vi "IMAQ FPGA Camera Link Data to Pixels 8 Tap 10-Bit.vi"(1 "Camera Link Data":T1) -> (0 "Pixels":u16[](array[numeric]))   [LabVIEW 2020]
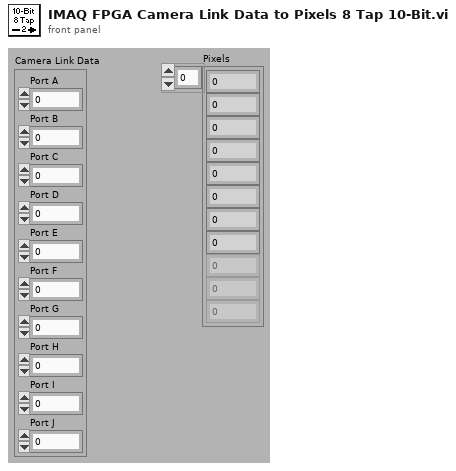
[diagram p1: front panel]
types:
  T1 = cluster{"Port A":u8, "Port B":u8, "Port C":u8, "Port D":u8, "Port E":u8, "Port F":u8, "Port G":u8, "Port H":u8, "Port I":u8, "Port J":u8}
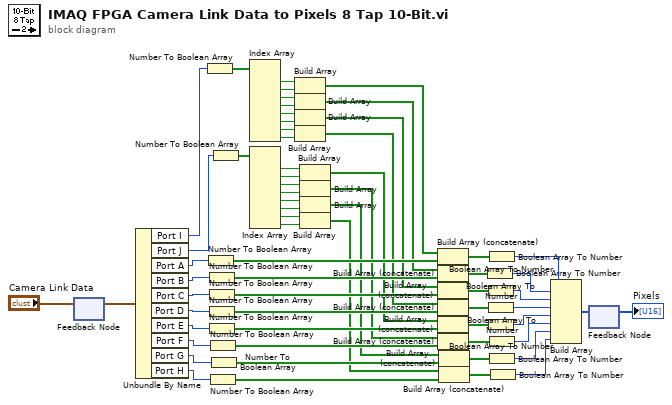
[diagram p0: block diagram]
diagram:
  n1 = feedback #1() -> (w1:T1)  [unwired: 1 in]
  n2 = feedback-in #1("Camera Link Data") -> ()
  n3 = Unbundle By Name(w1) -> ("Port I"=w52:u8, "Port J"=w51:u8, "Port A"=w64:u8, "Port B"=w61:u8, "Port C"=w58:u8, "Port D"=w56:u8, "Port E"=w49:u8, "Port F"=w47:u8, "Port G"=w18:u8, "Port H"=w7:u8)
  n4 = Number To Boolean Array(number=w52) -> (Boolean array=w40:bool[])
  n5 = Number To Boolean Array(number=w64) -> (Boolean array=w63:bool[])
  n6 = Number To Boolean Array(number=w61) -> (Boolean array=w60:bool[])
  n7 = Number To Boolean Array(number=w58) -> (Boolean array=w57:bool[])
  n8 = Number To Boolean Array(number=w56) -> (Boolean array=w55:bool[])
  n9 = Number To Boolean Array(number=w49) -> (Boolean array=w48:bool[])
  n10 = Number To Boolean Array(number=w47) -> (Boolean array=w26:bool[])
  n11 = Number To Boolean Array(number=w7) -> (Boolean array=w6:bool[])
  n12 = Number To Boolean Array(number=w18) -> (Boolean array=w14:bool[])
  n13 = Number To Boolean Array(number=w51) -> (Boolean array=w50:bool[])
  n14 = Index Array(array=w40) -> (element #1=w46:bool, element #2=w45:bool, element #3=w43:bool, element #4=w42:bool, element #5=w39:bool, element #6=w38:bool, element #7=w36:bool, element #8=w35:bool)  [unwired: 8 in]
  n15 = Index Array(array=w50) -> (element #1=w33:bool, element #2=w32:bool, element #3=w29:bool, element #4=w28:bool, element #5=w17:bool, element #6=w16:bool, element #7=w10:bool, element #8=w9:bool)  [unwired: 8 in]
  n16 = Build Array(w46, w45) -> (w44:bool[])
  n17 = Build Array(w43, w42) -> (w41:bool[])
  n18 = Build Array(w39, w38) -> (w37:bool[])
  n19 = Build Array(w36, w35) -> (w34:bool[])
  n20 = Build Array(w33, w32) -> (w31:bool[])
  n21 = Build Array(w29, w28) -> (w27:bool[])
  n22 = Build Array(w17, w16) -> (w15:bool[])
  n23 = Build Array(w10, w9) -> (w8:bool[])
  n24 = Build Array (concatenate)(w44, w63) -> (w62:bool[])
  n25 = Build Array (concatenate)(w41, w60) -> (w59:bool[])
  n26 = Build Array (concatenate)(w37, w57) -> (w54:bool[])
  n27 = Build Array (concatenate)(w34, w55) -> (w53:bool[])
  n28 = Build Array (concatenate)(w31, w48) -> (w30:bool[])
  n29 = Build Array (concatenate)(w27, w26) -> (w25:bool[])
  n30 = Build Array (concatenate)(w15, w14) -> (w13:bool[])
  n31 = Build Array (concatenate)(w8, w6) -> (w11:bool[])
  n32 = Boolean Array To Number(Boolean array=w59) -> (number=w23:u16)
  n33 = Boolean Array To Number(Boolean array=w54) -> (number=w22:u16)
  n34 = Boolean Array To Number(Boolean array=w53) -> (number=w21:u16)
  n35 = Boolean Array To Number(Boolean array=w30) -> (number=w20:u16)
  n36 = Boolean Array To Number(Boolean array=w62) -> (number=w24:u16)
  n37 = Boolean Array To Number(Boolean array=w25) -> (number=w19:u16)
  n38 = Boolean Array To Number(Boolean array=w13) -> (number=w12:u16)
  n39 = Boolean Array To Number(Boolean array=w11) -> (number=w5:u16)
  n40 = Build Array(w24, w23, w22, w21, w20, w19, w12, w5) -> (w4:u16[])
  n41 = feedback-in #2(w4) -> ()
  n42 = feedback #2() -> (→"Pixels":u16[])  [unwired: 1 in]
